vi "DisplaySettings 2 INI Section.vi"(8 "error in (no error)":errorcluster, 10 "Display settings":T2={"Min. Thresh."=0.0, "X"=0.0, "Y"=0.0, "ShowLineout"=FALSE, "ScaleParts"=10, "ShowLegende"=FALSE, "Target Cross"=FALSE, "Centroid Cross"=FALSE, "Target color"=16777226, "Centroid color"=16711680, "calibr. µm/px"=0.0}, 11 "refnum in":T1) -> (0 "error out":errorcluster, 3 "refnum out":T1)   [LabVIEW 2014, in "HIJ Vision Display.lvlib" / "HIJ Vision Display.lvclass"]
uses:
  HIJ Vision Display.lvclass
  DisplaySettings.ctl
  <vilib>/Utility/config.llb/Config Data RefNum.ctl
  <vilib>/Utility/config.llb/Write Key (Double).vi
  <vilib>/Utility/config.llb/NI_LVConfig.lvlib
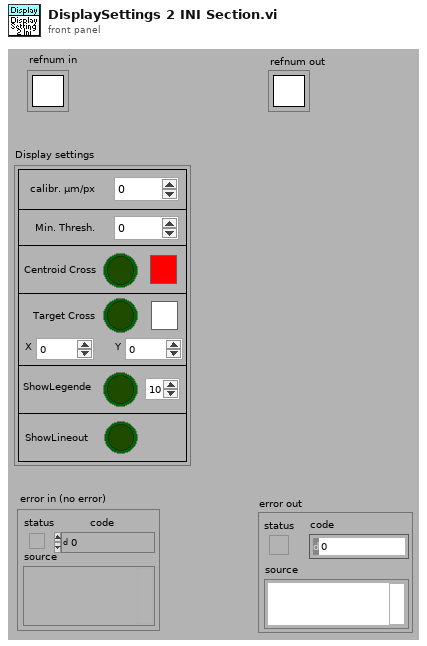
[diagram p1: front panel]
types:
  T1 = typedef "NI_LVConfig.lvlib/Config Data RefNum.ctl" = refnum<k1>
  T2 = typedef "HIJ Vision Display.lvlib/HIJ Vision Display.lvclass/DisplaySettings.ctl" = cluster{"Min. Thresh.":sgl, "X":dbl, "Y":dbl, "ShowLineout":bool, "ScaleParts":i32, "ShowLegende":bool, "Target Cross":bool, "Centroid Cross":bool, "Target color":u32, "Centroid color":u32, "calibr. µm/px":sgl[unit]}
  T3 = enum16{"fractional", "engineering", "exponential"}
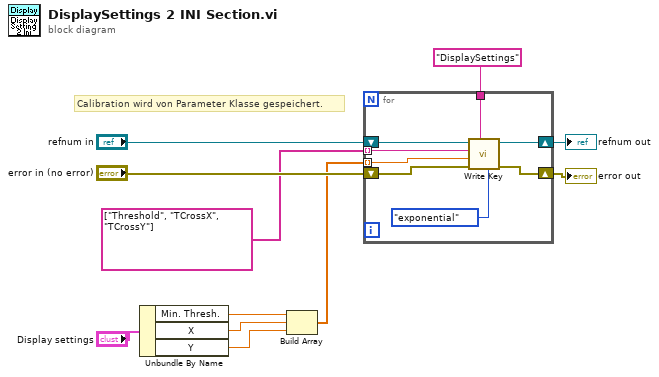
[diagram p0: block diagram]
diagram:
  # "Calibration wird von Parameter Klasse gespeichert."
  n1 = Unbundle By Name("Display settings") -> ("Min. Thresh."=w7:sgl, "X"=w6:dbl, "Y"=w5:dbl)
  n2 = Build Array(w7, w6, w5) -> (w2:dbl[])
  n3 = for {
    tunnel: "DisplaySettings" ("section") -> [w17]
    tunnel: w2 -> [w14] mode=indexing
    shift-right: [w15] -> w3
    shift-left: "error in (no error)" -> [w16]
    tunnel: string[] ["Threshold", "TCrossX", "TCrossY"] -> [w13] mode=indexing
    shift-right: [w18] -> w9
    shift-left: "refnum in" -> [w19]
    n4 = call-poly <vilib>:"Write Key.vi"("format (fractional)"=T3."exponential", "section"=w17, "error in (no error)"=w16, "value"=w14, "key"=w13, "refnum"=w19) -> ("error out"=w15:errorcluster, "refnum out"=w18:T1)  [unwired: 3 in, 1 out]
  }
  "refnum out" <- w9
  "error out" <- w3
